vi "SimpleVisionAlign.vi"(8 "Manual Turn":dbl, 9 "Target Offset":dbl=7.029609680175781, 10 "Gyro Angle":dbl=-0.01, 11 "Throttle":dbl=0.0031496062992125984) -> (2 "Right Power":dbl=-0.06388000338096318, 3 "Left Power":dbl=0.07017921597938838)   [LabVIEW 2018]
uses:
  <vilib>/addons/control/pid/pid.llb/PID (DBL).vi
  <vilib>/addons/control/pid/NI_PID_pid.lvlib
panel:
  out "Waveform Chart":dbl(graph)
  in  "MinTurn":dbl=0.06 format="%#_13g"
  in  "Automatic Throttle":dbl
  in  "Manual Turn Divisor":dbl=5.0
  in  "PID gains":T1={"proportional gain (Kc)"=0.001, "integral time (Ti, min)"=0.0, "derivative time (Td, min)"=0.001} {"derivative time (Td, min)" format="%.5f"; "integral time (Ti, min)" format="%.3f"; "proportional gain (Kc)" format="%.3f"}
  in  "output range":cluster{"output high":dbl, "output low":dbl}={"output high"=0.4, "output low"=-0.4} {"output low" format="%.2f"; "output high" format="%.2f"}
  in  "Latency Compensator":i32
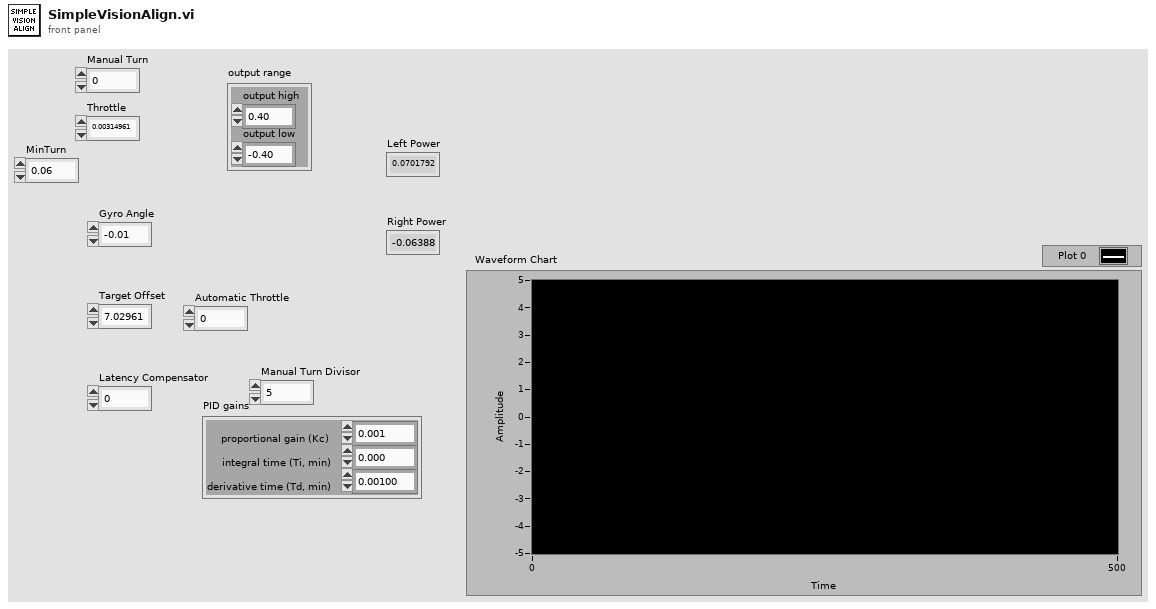
[diagram p1: front panel]
types:
  T1 = cluster{"proportional gain (Kc)":dbl, "integral time (Ti, min)":dbl, "derivative time (Td, min)":dbl}
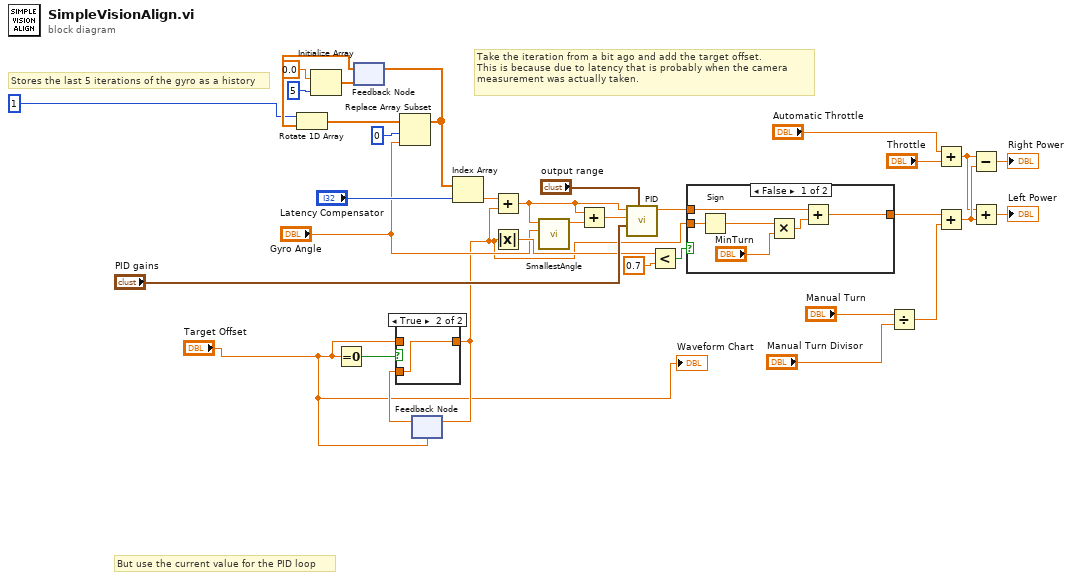
[diagram p0: block diagram]
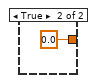
[diagram p3: hidden frame]
diagram:
  # "But use the current value for the PID loop"
  # "Take the iteration from a bit ago and add the target offset.\nThis is because due to latency that is probably when the camera\nmeasurement was actually taken."
  # "Stores the last 5 iterations of the gyro as a history"
  n1 = Initialize Array(0.0 ("element"), 5 ("dimension size")) -> (w27:dbl[])
  n2 = Equal To 0?(x="Target Offset") -> (x = 0?=w4:bool)
  n3 = feedback #1(w27) -> (w24:dbl[])
  n4 = Rotate 1D Array(1:w24, 2:1 ("n")) -> (0:w22:dbl[])
  n5 = Replace Array Subset(array=w22, new element="Gyro Angle", index=0) -> (w20:dbl[])
  n6 = feedback-in #1(w20) -> ()
  n7 = feedback #2("Target Offset") -> (w3:dbl)
  n8 = case shown="True" w4 {
    tunnel: "Target Offset" -> [w35 _]
    tunnel: [w35 w36] -> w2
    tunnel: w3 -> [_ w36]
    frame False {
    }
    frame True {
    }
  }
  n9 = feedback-in #2(w2) -> ()
  n10 = Index Array(array=w20, index="Latency Compensator") -> (element=w18:dbl)
  n11 = Add(x=w18, y=w2) -> (x+y=w29:dbl)
  n12 = Absolute Value(x=w2) -> (abs(x)=w6:dbl)
  n13 = call "SmallestAngle.vi"("Angle B"="Gyro Angle", "Angle A"=w29) -> ("Smallest A to B"=w30:dbl)  [unwired: 9 in]
  n14 = Add(x=w29, y=w30) -> (x+y=w28:dbl)
  n15 = call-poly <vilib>:"PID.vi"("output range"="output range", "PID gains"="PID gains", "process variable"=w28, "setpoint"=w29) -> ("output"=w8:dbl)  [unwired: 6 in, 1 out]
  n16 = Less?(x=w6, y=0.7) -> (x < y?=w9:bool)
  n17 = case shown="False" w9 {
    tunnel: w8 -> [w40 _]
    tunnel: [w38 0.0 ("y")] -> w7
    tunnel: w2 -> [w37 _]
    frame False {
      n18 = Sign(1:w37) -> (0:w41:dbl)
      n19 = Multiply(x=w41, y="MinTurn") -> (x*y=w39:dbl)
      n20 = Add(x=w40, y=w39) -> (x+y=w38:dbl)
    }
    frame True {
    }
  }
  n21 = Divide(x="Manual Turn", y="Manual Turn Divisor") -> (x/y=w15:dbl)
  n22 = Add(x="Automatic Throttle", y="Throttle") -> (x+y=w12:dbl)
  n23 = Add(x=w7, y=w15) -> (x+y=w14:dbl)
  n24 = Subtract(x=w12, y=w14) -> (x-y=→"Right Power":dbl)
  n25 = Add(x=w12, y=w14) -> (x+y=→"Left Power":dbl)
  "Waveform Chart" <- "Target Offset"
